vi "MSScript_Calc_CheckOP.vi"(5 "Operator in":ext[](array[numeric]), 7 "Operand in":ext[](array[numeric])) -> (0 "Cmd Error?":bool, 1 "Operator out":ext[](array[numeric]), 3 "Operand out":ext[](array[numeric]))   [LabVIEW 2018, in "MSScript.lvclass"]
uses:
  MSScript.lvclass
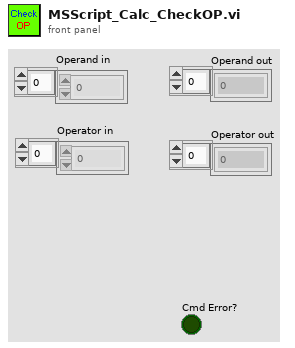
[diagram p1: front panel]
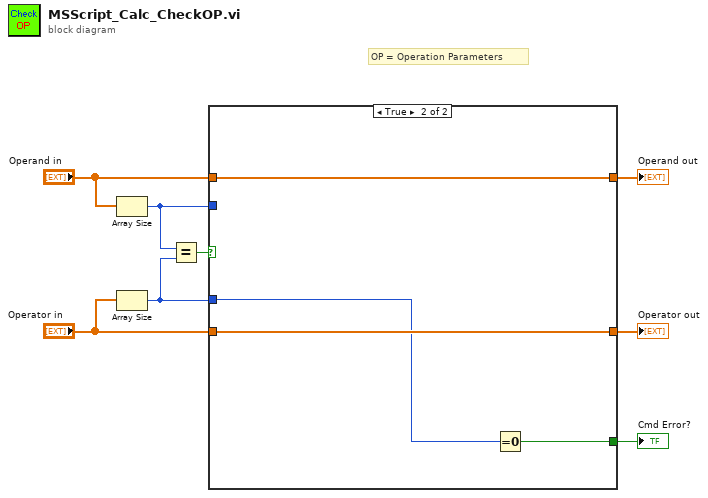
[diagram p0: block diagram]
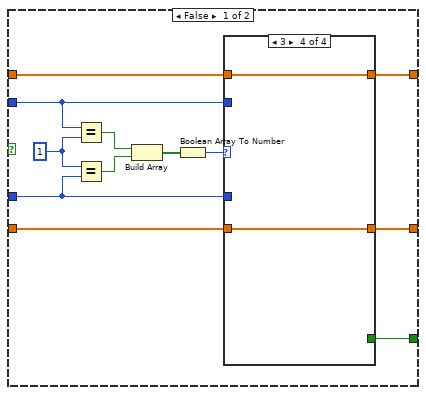
[diagram p2: hidden frame]
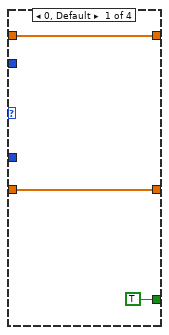
[diagram p3: hidden frame]
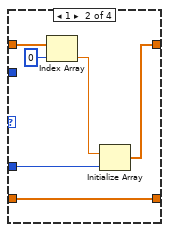
[diagram p4: hidden frame]
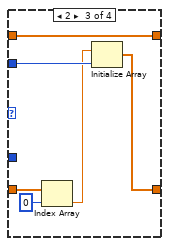
[diagram p5: hidden frame]
diagram:
  # "OP = Operation Parameters"
  n1 = Array Size(array="Operand in") -> (size(s)=w6:i32)
  n2 = Array Size(array="Operator in") -> (size(s)=w7:i32)
  n3 = Equal?(x=w6, y=w7) -> (x = y?=w8:bool)
  n4 = case shown="True" w8 {
    tunnel: w7 -> [w9 w38]
    tunnel: w6 -> [w15 _]
    tunnel: "Operator in" -> [w20 w40]
    tunnel: [w19 w39] -> w1
    tunnel: [w18 w40] -> w2
    tunnel: [w17 w41] -> w3
    tunnel: "Operand in" -> [w16 w41]
    frame False {
      w14 = 1 ("y")
      n5 = Equal?(x=w15, y=w14) -> (x = y?=w13:bool)
      n6 = Equal?(x=w14, y=w9) -> (x = y?=w12:bool)
      n7 = Build Array(w13, w12) -> (w11:bool[])
      n8 = Boolean Array To Number(Boolean array=w11) -> (number=w10:u32)
      n9 = case shown="3" w10 {
        tunnel: w15 -> [_ _ w33 _]
        tunnel: w20 -> [w23 w29 w35 w36]
        tunnel: [w23 w29 w31 w36] -> w18
        tunnel: [TRUE _ _ _] -> w19
        tunnel: [w21 w24 w30 w37] -> w17
        tunnel: w16 -> [w21 w25 w30 w37]
        tunnel: w9 -> [_ w26 _ _]
        frame 0, Default {
        }
        frame 1 {
          n10 = Index Array(array=w25, index=0) -> (element=w27:ext)
          n11 = Initialize Array(w27, w26) -> (w24:ext[])
        }
        frame 2 {
          n12 = Index Array(array=w35, index=0) -> (element=w32:ext)
          n13 = Initialize Array(w32, w33) -> (w31:ext[])
        }
        frame 3 {
        }
      }
    }
    frame True {
      n14 = Equal To 0?(x=w38) -> (x = 0?=w39:bool)
    }
  }
  "Operand out" <- w3
  "Operator out" <- w2
  "Cmd Error?" <- w1
